vi "Simple Reader.vi"(8 "error in (no error)":errorcluster, 11 "Keithley Driver in":refnum<class "Keithley Driver.lvclass">) -> (0 "error out":errorcluster, 2 "Signals":dbl[](array[numeric]), 3 "Keithley Driver out":refnum<class "Keithley Driver.lvclass">)   [LabVIEW 2018, in "Keithley Driver.lvclass"]
uses:
  Keithley Driver.lvclass
  C:/GitHub/NHMFL_Core/Libraries/Instruments/VISA Instrument/VISA Instrument.lvclass
  VISA Instrument/VISA Instrument.lvclass/VISA Instrument.ctl
  Keithley Driver.lvclass/Keithley Driver.ctl
  VISA Instrument/Read VISA resource.vi
  Read Auto-init.vi
  VISA Instrument/Write VISA resource.vi
  Read Keithley user configuration.vi
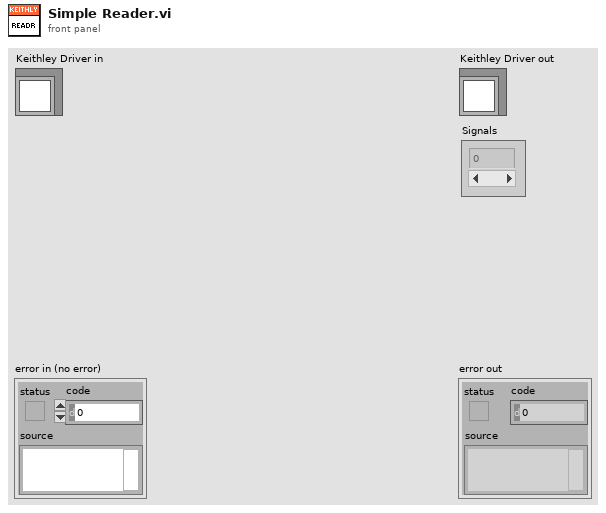
[diagram p1: front panel]
types:
  T1 = typedef "Keithley Meter Parameters.ctl" = cluster{"Range (-1: auto)":dbl, "Integration Time (NPLCs)":dbl, "Function":T2, "W Offset comp":bool, "4-wire W":bool, "Scale":dbl, "Offset":dbl}
  T2 = typedef "KeithleyMeter Function.ctl" = enum16{"VOLTAGE", "CURRENT", "RESISTANCE"}
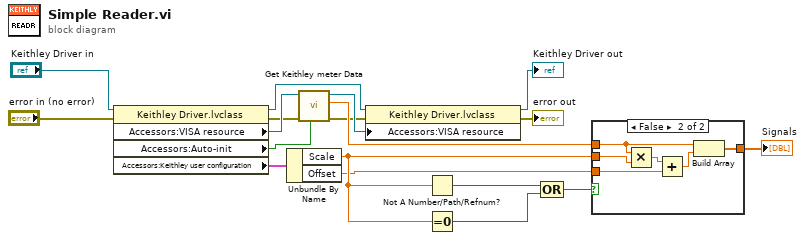
[diagram p0: block diagram]
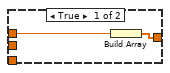
[diagram p2: hidden frame]
diagram:
  n1 = property class="Keithley Driver.lvclass"(reference="Keithley Driver in", error in="error in (no error)") -> (reference out=w18:refnum<class "Keithley Driver.lvclass">, error out=w9:errorcluster, "Accessors:VISA resource"=w13:refnum<visa-resource-name>, "Accessors:Auto-init"=w7:bool, "Accessors:Keithley user configuration"=w6:T1)
  n2 = Unbundle By Name(w6) -> ("Scale"=w2:dbl, "Offset"=w1:dbl)
  n3 = call "Get Keithley meter Data.vi"("INIT after?"=w7, "error in (no error)"=w9, "VISA Resource Name"=w13) -> ("error out"=w8:errorcluster, "Data"=w11:dbl, "VISA Resource Name Out"=w12:refnum<visa-resource-name>)  [unwired: 6 in]
  n4 = property class="Keithley Driver.lvclass"(reference=w18, error in=w8, "Accessors:VISA resource"=w12) -> (reference out=→"Keithley Driver out":refnum<class "Keithley Driver.lvclass">, error out=→"error out":errorcluster)
  n5 = Not A Number/Path/Refnum?(number/path/refnum=w2) -> (NaN/Path/Refnum?=w5:bool)
  n6 = Equal To 0?(x=w2) -> (x = 0?=w4:bool)
  n7 = Compound Arithmetic op=OR(w5, w4) -> (w3:bool)
  n8 = case shown="False" w3 {
    tunnel: w11 -> [w20 w25]
    tunnel: [w19 w26] -> w10
    tunnel: w2 -> [_ w24]
    tunnel: w1 -> [_ w21]
    frame True {
      n9 = Build Array(w20) -> (w19:dbl[])
    }
    frame False {
      n10 = Multiply(x=w25, y=w24) -> (x*y=w22:dbl)
      n11 = Add(x=w22, y=w21) -> (x+y=w23:dbl)
      n12 = Build Array(w25, w23) -> (w26:dbl[])
    }
  }
  "Signals" <- w10
